vi "Draw Legend Cluster.vi"(8 "error in (no error)":errorcluster, 9 "Plot Area Ref":refnum<vi>, 10 "Number Of Rows":i32, 11 "2D Error Bar.lvclass in":refnum<class "2D Error Bar.lvclass">) -> (0 "error out":errorcluster, 1 "Legend Cluster":T1(array[cluster]), 3 "2D Error Bar.lvclass out":refnum<class "2D Error Bar.lvclass">)   [LabVIEW 2017, in "2D Error Bar.lvclass"]
uses:
  <vilib>/Math Plots/2D Math Plots/2D Error Bar/2D Error Bar/2D Error Bar.lvclass
  <vilib>/Math Plots/2D Math Plots/2D Error Bar/2D Error Bar/2D Error Bar.lvclass/2D Error Bar.ctl
  <vilib>/Math Plots/2D Math Plots/2D Error Bar/2D Error Bar/Typedef/2D Error Bar Property.ctl
  <vilib>/Math Plots/2D Math Plots/2D Plot/2D Plot/2D Plot.lvclass
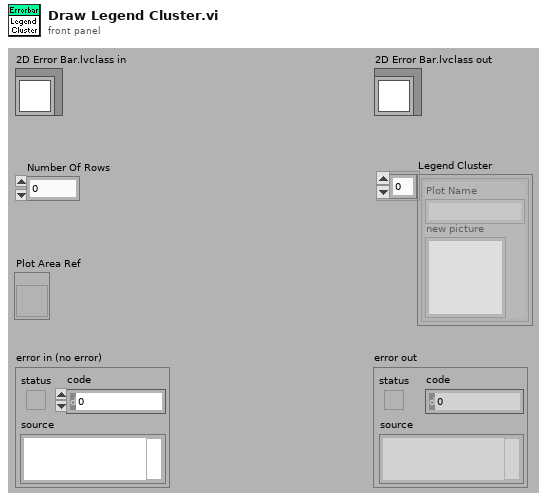
[diagram p1: front panel]
types:
  T1 = cluster{"Plot Name":string, "new picture":picture}[]
  T2 = typedef "2D Plot.lvclass/Plot Property Array.ctl" = T3[]
  T3 = typedef "2D Plot.lvclass/Plot Property.ctl" = cluster{"Bar Plot Style":u8, "DigitalLineStyle":u8, "TransitionLocation":u8, "Transition Type":u8, "Fill To":i16, "Fill/Pt. Color":u32, "Label Style":u8, "Line Style":u8, "Line Width":u8, "Plot Color":u32, "Plot Interpolation":u8, "Plot Name":string, "Point Style":u8, "Visible?":bool, "XScaleIdx":u32, "YScaleIdx":u32}
  T4 = typedef "2D Error Bar.lvclass/2D Error Bar Property Array.ctl" = T5[]
  T5 = typedef "2D Error Bar.lvclass/2D Error Bar Property.ctl" = cluster{"Marker Size":dbl, "Marker Line Style":u8, "Marker Line Width":u8, "Marker Color":u32, "Error Bar Interpolation":enum16{"Show Point", "Show Line", "Show Bar"}, "Error Mode":enum16{"Show Y Error", "Show X Error", "Show Both Error"}}
  T6 = cluster{"left":i16, "top":i16, "right":i16, "bottom":i16}
  T7 = cluster{"Width":u16, "Style":enum32{"Solid", "Dash", "Dot", "DashDot", "DashDotDot"}}
  T8 = cluster{"Plot Name":string, "new picture":picture}
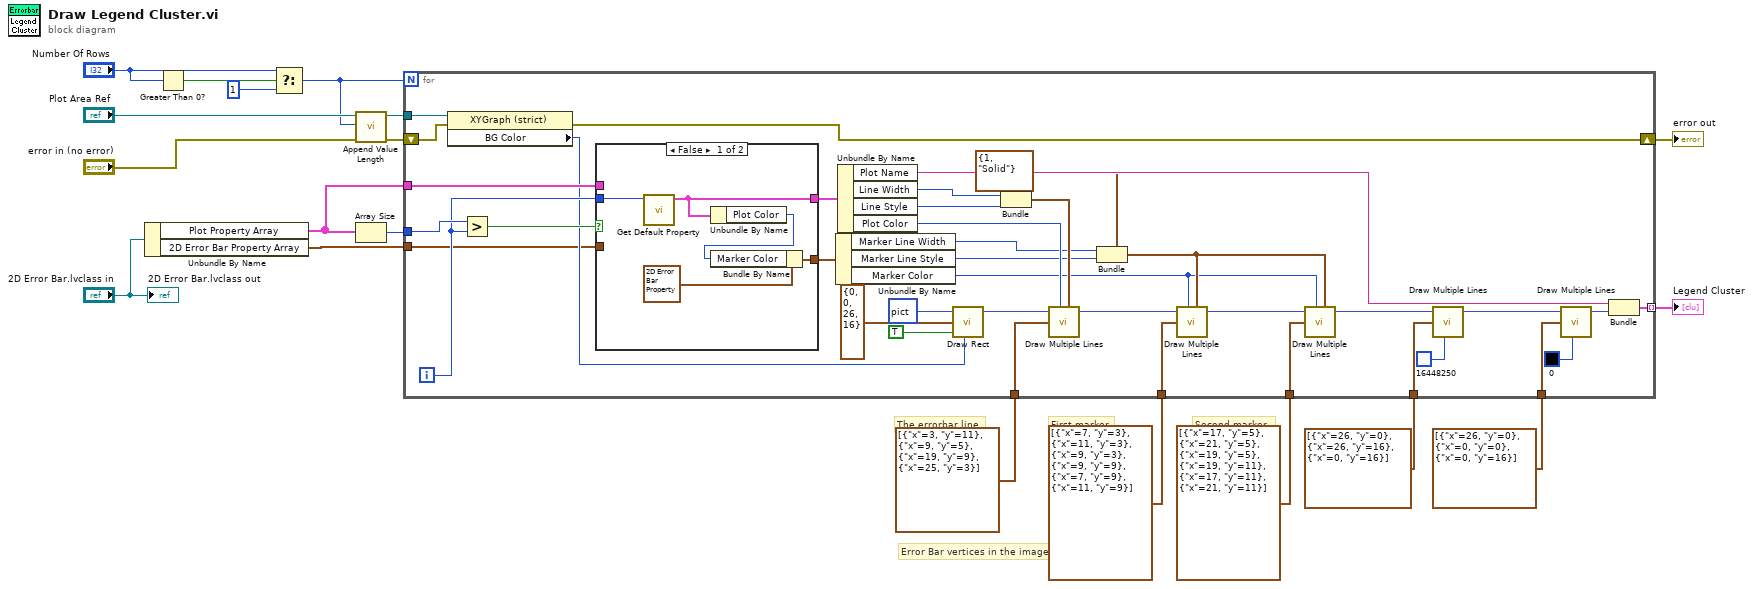
[diagram p0: block diagram]
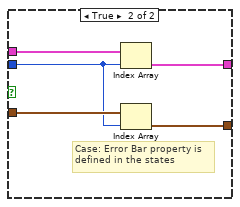
[diagram p2: hidden frame]
diagram:
  # "Second marker"
  # "First marker"
  # "The errorbar line"
  # "Error Bar vertices in the image"
  n1 = Unbundle By Name("2D Error Bar.lvclass in") -> ("Plot Property Array"=w14:T2, "2D Error Bar Property Array"=w1:T4)
  n2 = Greater Than 0?(x="Number Of Rows") -> (x > 0?=w18:bool)
  n3 = Select(t="Number Of Rows", s=w18, f=1) -> (s? t:f=w7:i32)
  n4 = call <vilib>:"Append Value Length.vi"("error in (no error)"="error in (no error)", "Expect Value Length"=w7, "Plot Area Ref In"="Plot Area Ref") -> ("error out"=w8:errorcluster, "Plot Area Ref Out"=w10:refnum<vi>)  [unwired: 1 in, 6 out]
  n5 = Array Size(array=w14) -> (size(s)=w15:i32)
  n6 = for {
    N: w7 -> [_]
    tunnel: w14 -> [w48]
    tunnel: [w52] -> w19 mode=indexing
    tunnel: w15 -> [w50]
    tunnel: w10 -> [w39]
    shift-right: [w20] -> w12
    shift-left: w8 -> [w38]
    tunnel: cluster{"x":i16, "y":i16}[] [{"x"=3, "y"=11}, {"x"=9, "y"=5}, {"x"=19, "y"=9}, {"x"=25, "y"=3}] ("line endpoints") -> [w36]
    tunnel: cluster{"x":i16, "y":i16}[] [{"x"=7, "y"=3}, {"x"=11, "y"=3}, {"x"=9, "y"=3}, {"x"=9, "y"=9}, {"x"=7, "y"=9}, {"x"=11, "y"=9}] ("line endpoints") -> [w35]
    tunnel: cluster{"x":i16, "y":i16}[] [{"x"=17, "y"=5}, {"x"=21, "y"=5}, {"x"=19, "y"=5}, {"x"=19, "y"=11}, {"x"=17, "y"=11}, {"x"=21, "y"=11}] ("line endpoints") -> [w34]
    tunnel: cluster{"x":i16, "y":i16}[] [{"x"=26, "y"=0}, {"x"=26, "y"=16}, {"x"=0, "y"=16}] ("line endpoints") -> [w33]
    tunnel: cluster{"x":i16, "y":i16}[] [{"x"=26, "y"=0}, {"x"=0, "y"=0}, {"x"=0, "y"=16}] ("line endpoints") -> [w32]
    tunnel: w1 -> [w30]
    i -> [w47]
    w28 = T7 {"Width"=1, "Style"=enum."Solid"} ("pen")
    n7 = property class="XYGraph (strict)"(reference=w39, error in=w38) -> (error out=w20:errorcluster, "BG Color"=w37:u32)  [unwired: 1 out]
    n8 = Greater?(x=w50, y=w47) -> (0:w49:bool)
    n9 = case shown="False" w49 {
      tunnel: w48 -> [_ w67]
      tunnel: w47 -> [w59 w64]
      tunnel: [w58 w66] -> w46
      tunnel: w30 -> [_ w65]
      tunnel: [w61 w63] -> w29
      frame False {
        n10 = call <vilib>:"Get Default Property.vi"("Index"=w59) -> ("Temporary Property"=w58:T3)  [unwired: 3 in, 7 out]
        n11 = Unbundle By Name(w58) -> ("Plot Color"=w60:u32)
        n12 = Bundle By Name(cluster=T5 {"Marker Size"=0.0, "Marker Line Style"=0, "Marker Line Width"=0, "Marker Color"=0, "Error Bar Interpolation"=enum."Show Point", "Error Mode"=enum."Show Y Error"} ("2D Error Bar Property"), "Marker Color"=w60) -> (w61:T5)
      }
      frame True {
        # "Case: Error Bar property is \ndefined in the states"
        n13 = Index Array(array=w67, index=w64) -> (element=w66:T3)
        n14 = Index Array(array=w65, index=w64) -> (element=w63:T5)
      }
    }
    n15 = Unbundle By Name(w29) -> ("Marker Line Width"=w27:u8, "Marker Line Style"=w26:u8, "Marker Color"=w24:u32)
    n16 = Unbundle By Name(w46) -> ("Plot Name"=w53:string, "Line Width"=w55:u8, "Line Style"=w54:u8, "Plot Color"=w45:u32)
    n17 = call <vilib>:"Draw Rect.vi"("picture"=picture data[5B], "rect"=T6 {"left"=0, "top"=0, "right"=26, "bottom"=16}, "fill?(F)"=TRUE, "color(black)"=w37) -> ("new picture"=w31:picture)  [unwired: 1 in, 4 out]
    n18 = Bundle(cluster=w28, "Width"=w55, "Style"=w54) -> (w44:T7)
    n19 = call <vilib>:"Draw Multiple Lines.vi"("picture"=w31, "line endpoints"=w36, "color(black)"=w45, "pen"=w44) -> ("new picture"=w23:picture)  [unwired: 1 in, 4 out]
    n20 = Bundle(cluster=w28, "Width"=w27, "Style"=w26) -> (w25:T7)
    n21 = call <vilib>:"Draw Multiple Lines.vi"("picture"=w23, "line endpoints"=w35, "color(black)"=w24, "pen"=w25) -> ("new picture"=w22:picture)  [unwired: 1 in, 4 out]
    n22 = call <vilib>:"Draw Multiple Lines.vi"("picture"=w22, "line endpoints"=w34, "color(black)"=w24, "pen"=w25) -> ("new picture"=w21:picture)  [unwired: 1 in, 4 out]
    n23 = call <vilib>:"Draw Multiple Lines.vi"("picture"=w21, "line endpoints"=w33, "color(black)"=u32 16448250) -> ("new picture"=w41:picture)  [unwired: 2 in, 4 out]
    n24 = call <vilib>:"Draw Multiple Lines.vi"("picture"=w41, "line endpoints"=w32, "color(black)"=u32 0) -> ("new picture"=w40:picture)  [unwired: 2 in, 4 out]
    n25 = Bundle("Plot Name"=w53, "new picture"=w40) -> (w52:T8)  [unwired: 1 out]
  }
  "Legend Cluster" <- w19
  "error out" <- w12
  "2D Error Bar.lvclass out" <- "2D Error Bar.lvclass in"
